vi "Generate Trace for New Time Delayed Message.vi"(9 "Message Name":string, 10 "Delivery Notifier":refnum<notifier>, 11 "Caller Details":T1) -> ()   [LabVIEW 2020, in "Actor Framework.lvlib"]
doc: "Generates a DETT User Generated Trace for a time-delayed message being created."
uses:
  Actor Framework.lvlib
  Time-Delayed Send Message/Time-Delay Override Options.ctl
  Support/TDM Registration Mode.ctl
  Support/Registration Mode.ctl
  Support/Localized Strings.vi
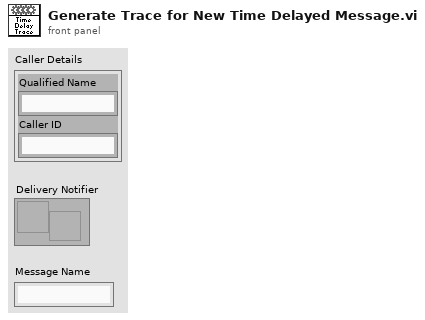
[diagram p1: front panel]
types:
  T1 = cluster{"Qualified Name":string, "Caller ID":string}
  T2 = typedef "Actor Framework.lvlib/TDM Registration Mode.ctl" = enum16{"Register TDM", "Get ID", "Get Notifier", "Deregister TDM"}
  T3 = typedef "Actor Framework.lvlib/Registration Mode.ctl" = enum16{"Register Actor", "Get ID", "Get Enqueuer", "Deregister Actor", "Get Update Event", "Get All Actors"}
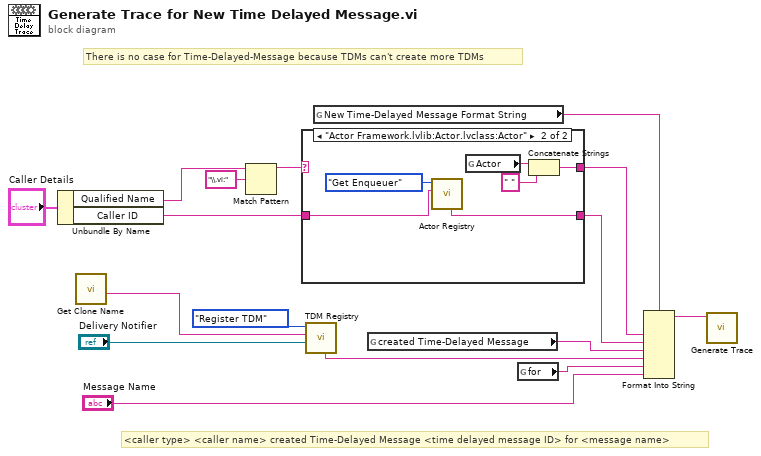
[diagram p0: block diagram]
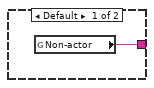
[diagram p2: hidden frame]
diagram:
  # "There is no case for Time-Delayed-Message because TDMs can't create more TDMs"
  # "<caller type> <caller name> created Time-Delayed Message <time delayed message ID> for <message name>"
  n1 = Unbundle By Name("Caller Details") -> ("Qualified Name"=w7:string, "Caller ID"=w6:string)
  n2 = call "Get Clone Name.vi"() -> ("Clone ID"=w2:string)  [unwired: 10 in, 1 out]
  n3 = Match Pattern(string=w7, regular expression="\\.vi:") -> (before substring=w16:string)  [unwired: 1 in, 3 out]
  n4 = case shown="\"Actor Framework.lvlib:Actor.lvclass:Actor\"" w16 {
    tunnel: [w17 w20] -> w15
    tunnel: [_ w21] -> w13
    tunnel: w6 -> [_ w18]
    frame Default {
      n5 = global read "Localized Strings.vi" "Non-actor"() -> (w17:string)
    }
    frame "Actor Framework.lvlib:Actor.lvclass:Actor" {
      n6 = call "Actor Registry.vi"("Actor ID"=w18, "Action"=Registration_Mode."Get Enqueuer") -> ("Actor Alias out"=w21:string)  [unwired: 5 in, 4 out]
      n7 = global read "Localized Strings.vi" "Actor"() -> (w22:string)
      n8 = Concatenate Strings(w22, " " ("string")) -> (w20:string)
    }
  }
  n9 = call "TDM Registry.vi"("Delivery Notifier"="Delivery Notifier", "TDM ID"=w2, "Action"=TDM_Registration_Mode."Register TDM") -> ("TDM Alias Out"=w4:string)  [unwired: 4 in, 4 out]
  n10 = global read "Localized Strings.vi" "New Time-Delayed Message Format String"() -> (w12:string)
  n11 = global read "Localized Strings.vi" "created Time-Delayed Message"() -> (w11:string)
  n12 = global read "Localized Strings.vi" "for"() -> (w10:string)
  n13 = Format Into String(format string=w12, w15, w13, w11, w4, w10, "Message Name") -> (resulting string=w1:string)  [unwired: 2 in, 1 out]
  n14 = call "Generate Trace.vi"("String"=w1) -> ()  [unwired: 11 in]
